vi "Servo MSMT ET Delay.vi"(8 "error in (no error)":errorcluster, 11 "Servo MSMT in":refnum<class "Servo MSMT.lvclass">) -> (0 "error out":errorcluster, 3 "Servo MSMT out":refnum<class "Servo MSMT.lvclass">)   [LabVIEW 2018, in "Servo MSMT.lvlib" / "Servo MSMT.lvclass"]
uses:
  Servo MSMT.lvclass
  C:/Sequence Automation/Plugins/Measurement Interface.lvlibp/Measurement Interface.lvclass
  Plugins/Measurement Interface.lvlibp/Private Methods/Measurement Parameters/Read Measurement Parameters.vi
  Plugins/String Database.lvlibp/String Database.lvclass
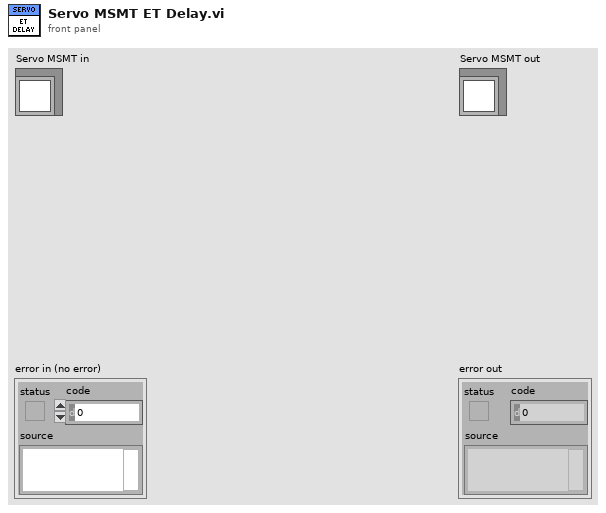
[diagram p1: front panel]
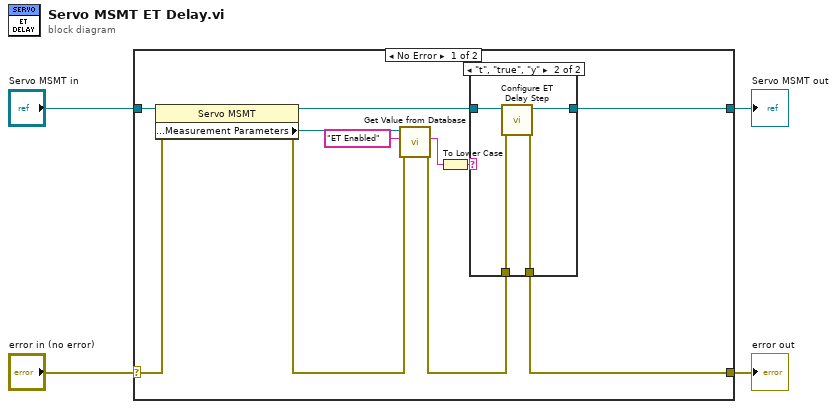
[diagram p0: block diagram]
diagram:
  n1 = case shown="No Error" "error in (no error)" {
    selector: "error in (no error)" -> [w15 w23]
    tunnel: [w9 w23] -> w3
    tunnel: [w7 w22] -> w1
    tunnel: "Servo MSMT in" -> [w14 w22]
    frame No Error {
      n2 = property class="Servo MSMT"(reference=w14, error in=w15) -> (reference out=w8:refnum<class "Servo MSMT.lvclass">, error out=w12:errorcluster, "Protected Methods:Measurement Parameters"=w13:refnum<class "String Database.lvclass">)
      n3 = call "Get Value from Database.vi"("error in (no error)"=w12, "Entry Name"="ET Enabled", "Message in"=w13) -> ("error out"=w11:errorcluster, "Entry Value"=w6:string)  [unwired: 5 in, 2 out]
      n4 = To Lower Case(string=w6) -> (all lower case string=w5:string)
      n5 = case shown="\"t\", \"true\", \"y\"" w5 {
        tunnel: w11 -> [w16 w21]
        tunnel: [w16 w20] -> w9
        tunnel: w8 -> [w17 w19]
        tunnel: [w17 w18] -> w7
        frame "False", Default {
        }
        frame "t", "true", "y" {
          n6 = call "Configure ET Delay Step.vi"("error in (no error)"=w21, "Servo MSMT in"=w19) -> ("error out"=w20:errorcluster, "Servo MSMT out"=w18:refnum<class "Servo MSMT.lvclass">)  [unwired: 8 in]
        }
      }
    }
    frame Error {
    }
  }
  "error out" <- w3
  "Servo MSMT out" <- w1
